vi "Volatus Config.vi"(8 "error in (no error)":errorcluster, 11 "VolatusAPI in":refnum<class "VolatusAPI.lvclass">) -> (0 "error out":errorcluster, 2 "Volatus Config":refnum<class "VolatusConfig.lvclass">, 3 "VolatusAPI out":refnum<class "VolatusAPI.lvclass">)   [LabVIEW 2020, in "Volatus.lvlib" / "VolatusAPI.lvclass"]
uses:
  VolatusAPI.lvclass
  VolatusAPI.lvclass/VolatusAPI.ctl
  VolatusConfig/VolatusConfig/VolatusConfig.lvclass
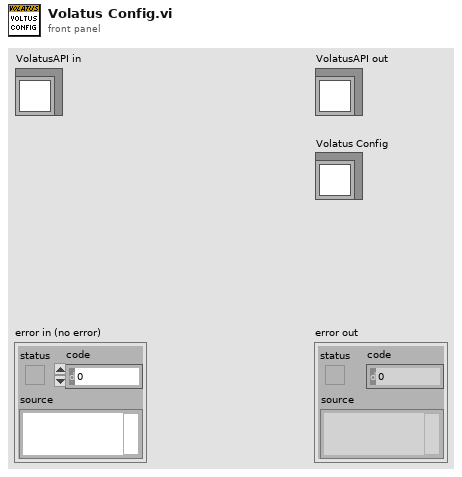
[diagram p1: front panel]
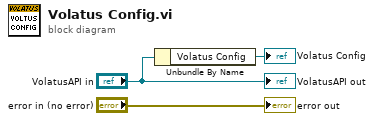
[diagram p0: block diagram]
diagram:
  n1 = Unbundle By Name("VolatusAPI in") -> ("Volatus Config"=→"Volatus Config":refnum<class "VolatusConfig.lvclass">)
  "error out" <- "error in (no error)"
  "VolatusAPI out" <- "VolatusAPI in"
